vi "jv_data_to_plot.vi"(8 "Data Array 2":dbl[][](array[numeric]), 11 "Data Array":dbl[][](array[numeric])) -> (3 "JV Curve":cluster{"Y":dbl[], "Y":dbl[]}[](graph))   [LabVIEW 2016]
panel:
  in  "Tab Control 4":enum32{"Page 1"}(tab)
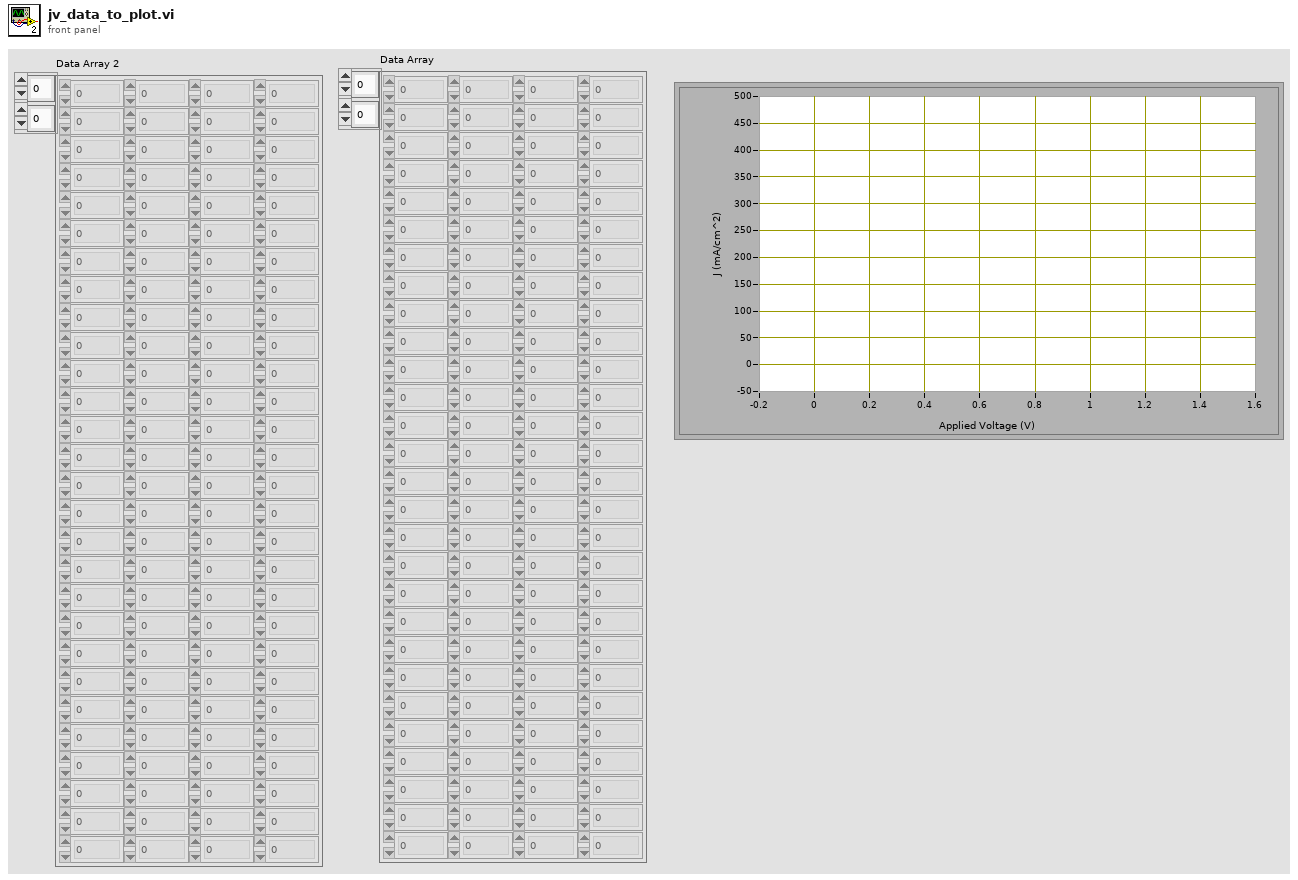
[diagram p1: front panel]
types:
  T1 = cluster{"Data Array 2":dbl[], "Data Array 2":dbl[]}
  T2 = cluster{"Data Array 2":dbl[], "Data Array 2":dbl[]}[]
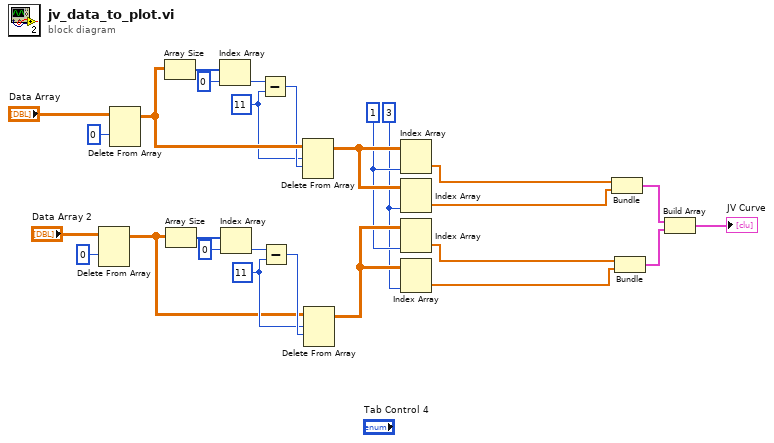
[diagram p0: block diagram]
diagram:
  w5 = 11 ("y")
  w11 = 11 ("y")
  w1 = 3
  w2 = 1
  n1 = Delete From Array(array="Data Array 2", index (row)=0) -> (array with subset deleted=w4:dbl[][])  [unwired: 2 in, 1 out]
  n2 = Delete From Array(array="Data Array", index (row)=0) -> (array with subset deleted=w14:dbl[][])  [unwired: 2 in, 1 out]
  n3 = Array Size(array=w14) -> (size(s)=w16:i32[])
  n4 = Array Size(array=w4) -> (size(s)=w9:i32[])
  n5 = Index Array(array=w16, index=0) -> (element=w13:i32)
  n6 = Index Array(array=w9, index=0) -> (element=w7:i32)
  n7 = Subtract(x=w13, y=w11) -> (x-y=w12:i32)
  n8 = Subtract(x=w7, y=w5) -> (x-y=w6:i32)
  n9 = Delete From Array(array=w14, length=w11, index (row)=w12) -> (array with subset deleted=w10:dbl[][])  [unwired: 1 in, 1 out]
  n10 = Delete From Array(array=w4, length=w5, index (row)=w6) -> (array with subset deleted=w3:dbl[][])  [unwired: 1 in, 1 out]
  n11 = Index Array(array=w10, index (col)=w2) -> (element=w27:dbl[])  [unwired: 1 in]
  n12 = Index Array(array=w10, index (col)=w1) -> (element=w22:dbl[])  [unwired: 1 in]
  n13 = Index Array(array=w3, index (col)=w2) -> (element=w26:dbl[])  [unwired: 1 in]
  n14 = Index Array(array=w3, index (col)=w1) -> (element=w21:dbl[])  [unwired: 1 in]
  n15 = Bundle("Data Array"=w27, "Data Array"=w22) -> (w24:cluster{"Data Array":dbl[], "Data Array":dbl[]})  [unwired: 1 in]
  n16 = Bundle("Data Array 2"=w26, "Data Array 2"=w21) -> (w25:T1)  [unwired: 1 in]
  n17 = Build Array(w24, w25) -> (→"JV Curve":T2)
